vi "ExSubCloseExperimentEm.vi"(1 "error in (no error)":errorcluster, 2 "Handles In":T1) -> (0 "error out":errorcluster)   [LabVIEW 2010]
panel:
  # "ExSubCloseExperimentEM:\nThis Sub VI closes an experiment."
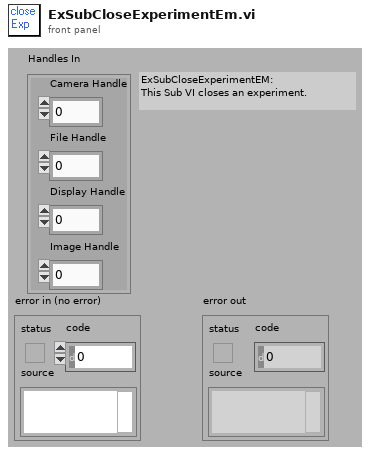
[diagram p1: front panel]
types:
  T1 = cluster{"Camera Handle":u32, "File Handle":u32, "Display Handle":u32, "Image Handle":u32}
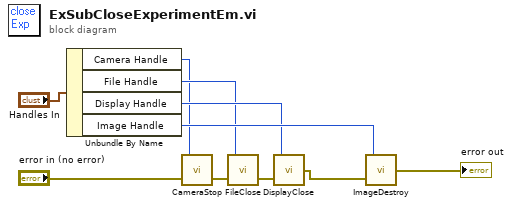
[diagram p0: block diagram]
diagram:
  n1 = Unbundle By Name("Handles In") -> ("Camera Handle"=w3:u32, "File Handle"=w6:u32, "Display Handle"=w7:u32, "Image Handle"=w8:u32)
  n2 = call <userlib>:"CameraStop.vi"("error in"="error in (no error)", "Camera Handle"=w3) -> ("error out"=w5:errorcluster)  [unwired: 1 out]
  n3 = call <userlib>:"FileClose.vi"("error in"=w5, "File Handle"=w6) -> ("error out"=w9:errorcluster)
  n4 = call <userlib>:"DisplayClose.vi"("error in"=w9, "Display Handle"=w7) -> ("error out"=w2:errorcluster)
  n5 = call <userlib>:"ImageDestroy.vi"("error in"=w2, "Data handle"=w8) -> ("error out"=→"error out":errorcluster)
